vi "_AllThingsBS.vi"   [LabVIEW 2012]
uses:
  <vilib>/NXT/LegoClasses/BotSpeak/BotSpeak.lvclass
  <vilib>/NXT/LegoClasses/BrickManagers/BotSpeakManager/BotSpeakManager.lvclass
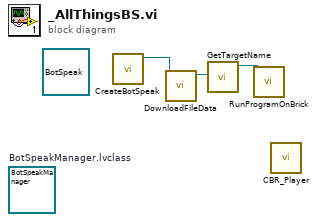
[diagram p0: block diagram]
diagram:
  (unwired) refnum<class "BotSpeakManager.lvclass"> refnum  # BotSpeakManager.lvclass
  (unwired) refnum<class "BotSpeak.lvclass"> refnum ("BotSpeak.lvclass")
  n1 = call <vilib>:"CreateBotSpeak.vi"() -> ("VIA.lvclass"=w3:refnum<class "BotSpeak.lvclass">)  [unwired: 11 in]
  n2 = call-dynamic "DownloadFileData.vi"("VIA in"=w3) -> ("VIA out"=w2:refnum<class "BotSpeak.lvclass">)  [unwired: 7 in, 3 out]
  n3 = call-dynamic "GetTargetName.vi"("VIA in"=w2) -> ("VIA out"=w1:refnum<class "BotSpeak.lvclass">)  [unwired: 8 in, 2 out]
  n4 = call-dynamic "RunProgramOnBrick.vi"("VIA in"=w1) -> ()  [unwired: 9 in, 2 out]
  n5 = call <vilib>:"CBR_Player.vi"() -> ()  [unwired: 12 in]
